vi "Output Message.vi"(0 "Message Expression in":string, 1 "Sequence Context In":refnum<k7>, 5 "Category Expression in":string, 7 "Severity Expression in":string, 9 "Message Severity in":u16(ring) caption="Message Severity" items=["Information", "Warning", "Error"], 11 "Use Severity Expression ? in":bool) -> (4 "Message Expression out":string, 6 "Category Expression out":string, 8 "Severity Expression out":string, 10 "Message Severity out":u16(ring) caption="Message Severity" items=["Information", "Warning", "Error"], 14 "error out":errorcluster, 15 "Use Severity Expression ? out":bool)   [LabVIEW 2020]
uses:
  <vilib>/addons/TestStand/_TSUtility.llb/TestStand - Start Modal Dialog (Sequence Context).vi
  <vilib>/addons/TestStand/_TSUtility.llb/TestStand - End Modal Dialog (Sequence Context).vi
panel:
  in  "Severity Option":T1(tab)
  in  "Message Severity":refnum<k7>(container)
  in  "Cancel":bool
  in  "OK":bool
  in  "Message Category":refnum<k7>(container)
  in  "Message String":refnum<k7>(container)
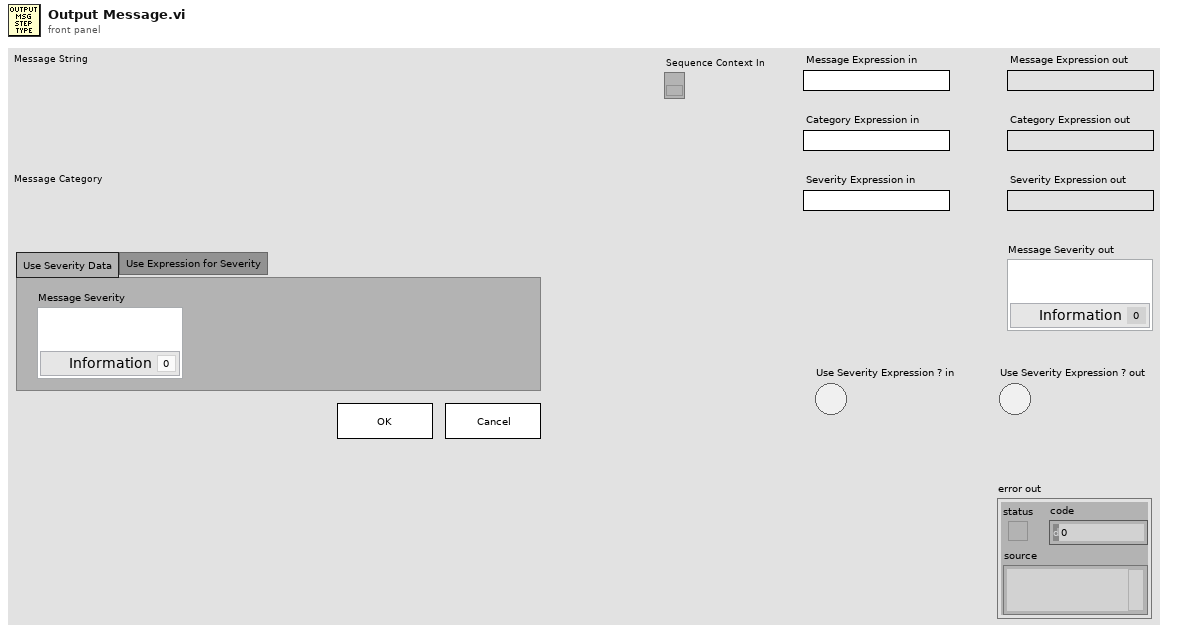
[diagram p1: front panel]
types:
  T1 = enum32{"Use Severity Data", "Use Expression for Severity"}
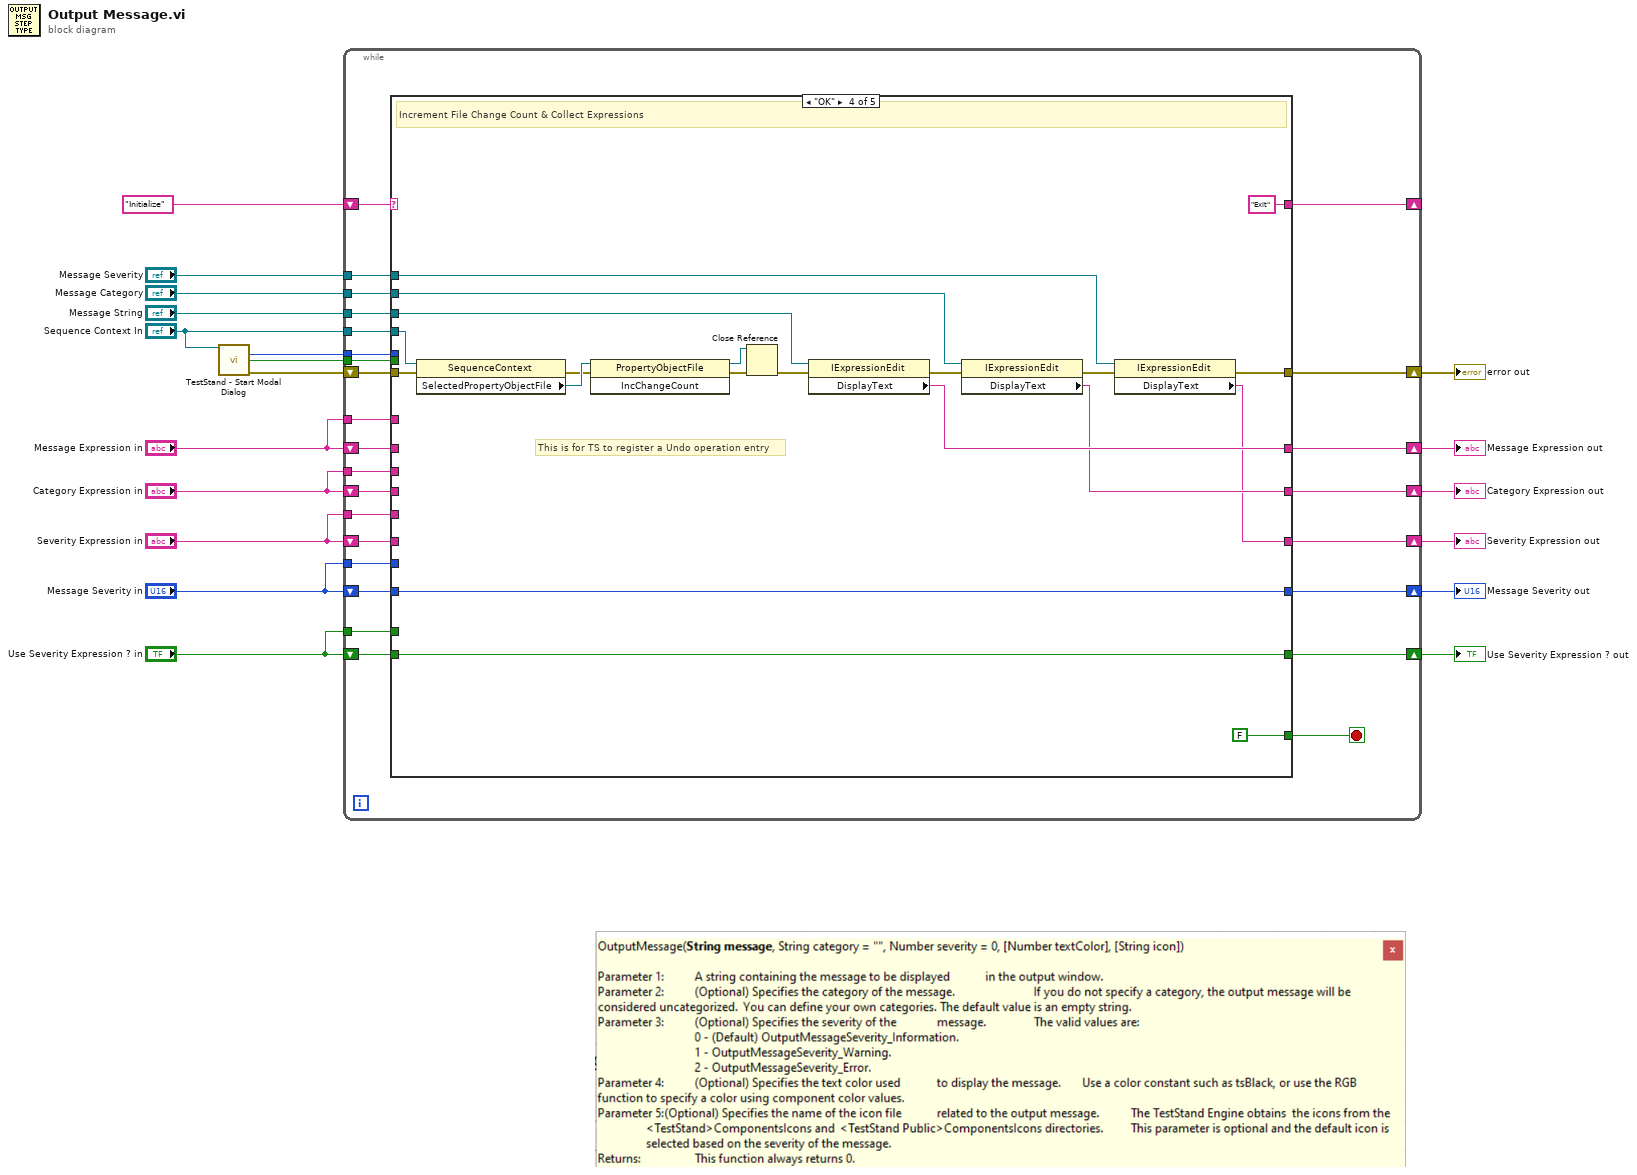
[diagram p0: block diagram]
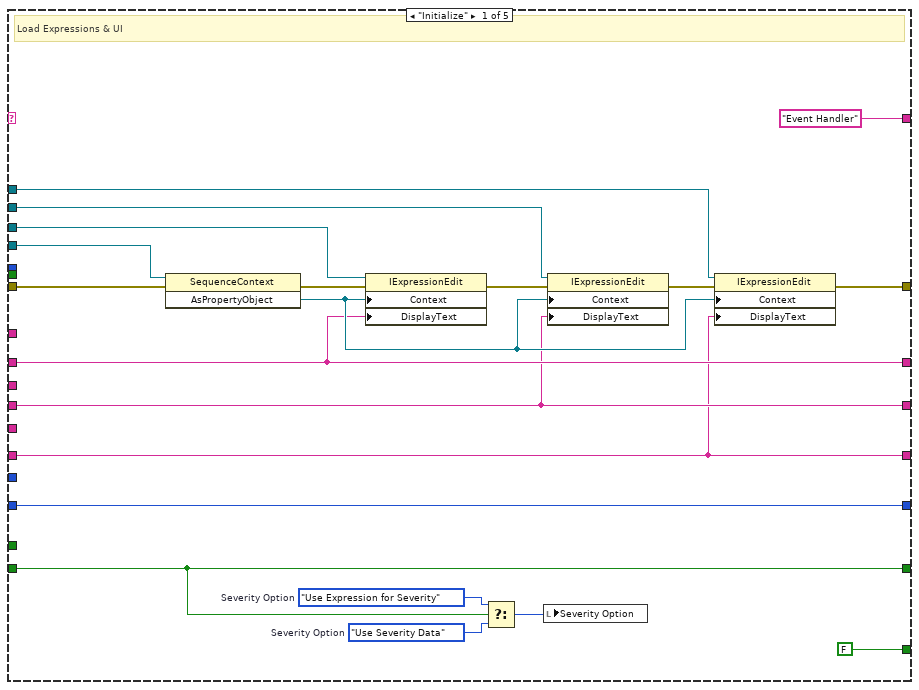
[diagram p2: hidden frame]
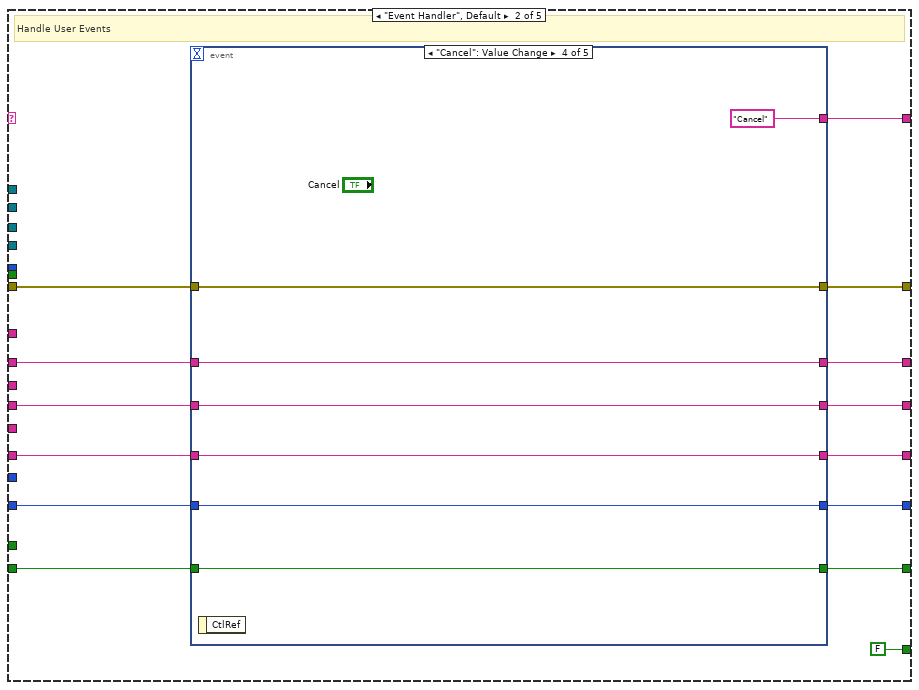
[diagram p3: hidden frame]
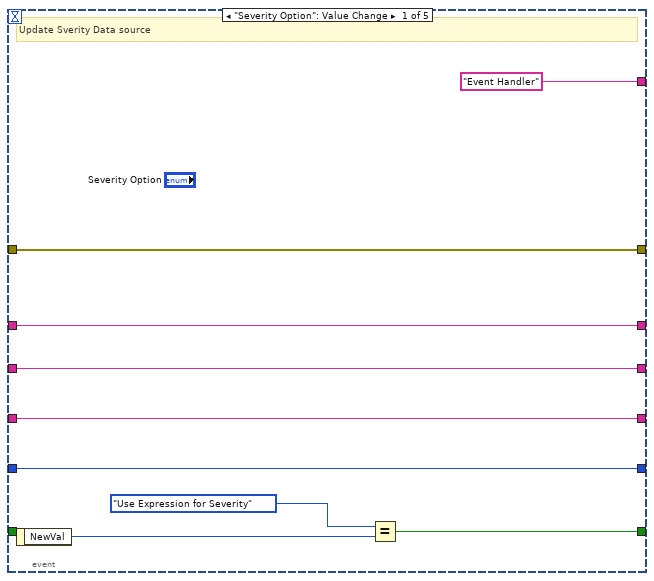
[diagram p4: hidden frame]
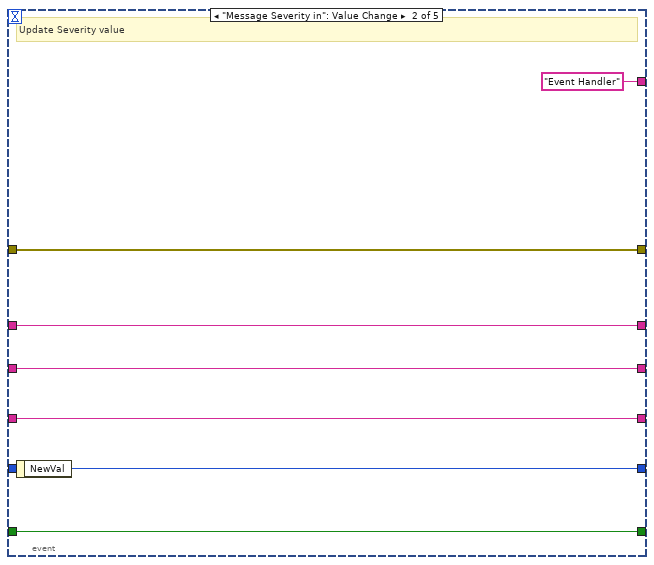
[diagram p5: hidden frame]
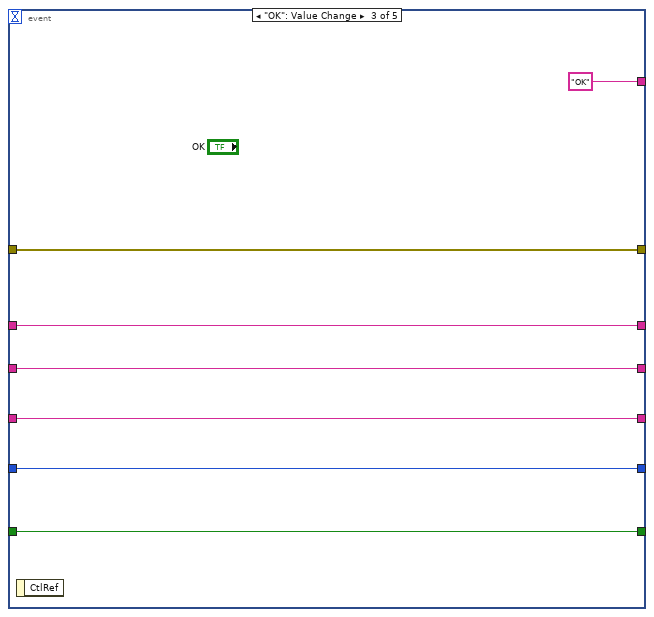
[diagram p6: hidden frame]
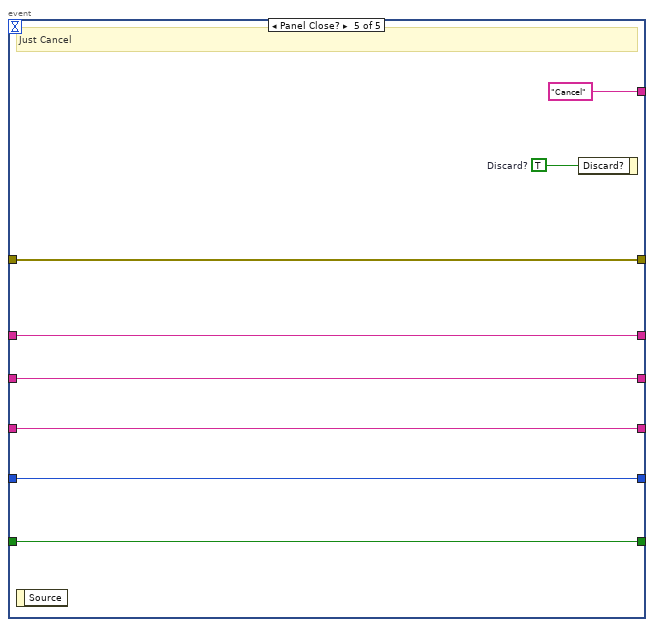
[diagram p7: hidden frame]
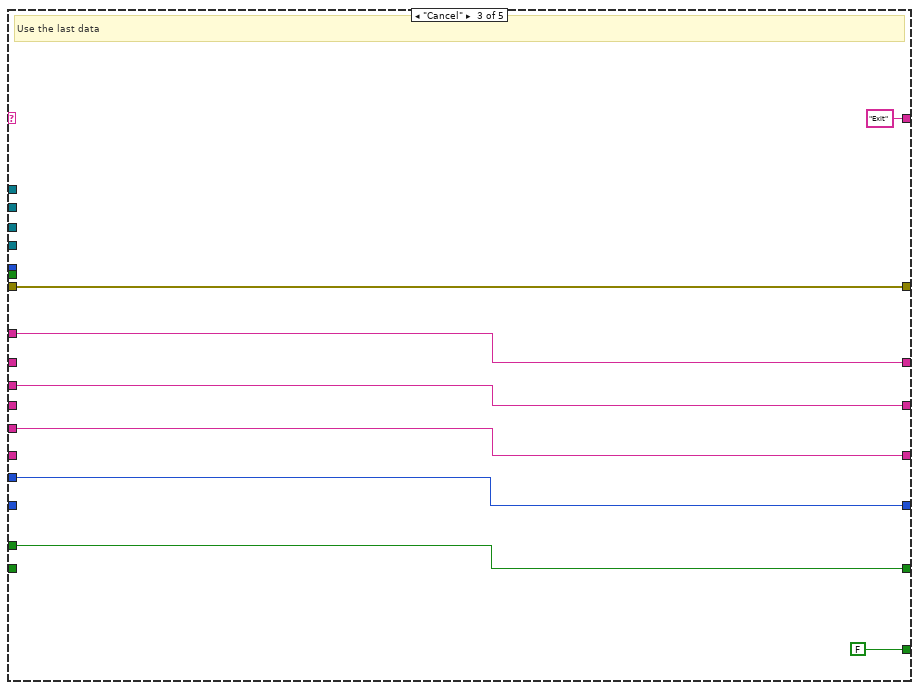
[diagram p8: hidden frame]
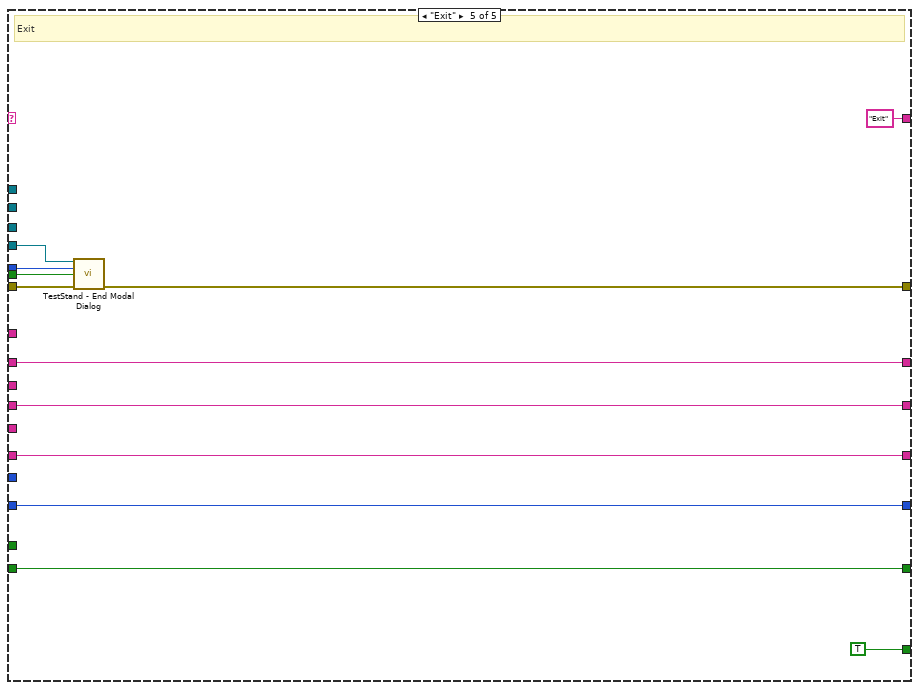
[diagram p9: hidden frame]
diagram:
  n1 = call-poly <vilib>:"TestStand - Start Modal Dialog.vi"("Sequence Context In"="Sequence Context In") -> ("Modal ID"=w2:i32, "VI Originally Open"=w1:bool, "error out"=w4:errorcluster)  [unwired: 10 in, 2 out]
  n2 = while {
    tunnel: "Sequence Context In" -> [w45]
    tunnel: "Message String" -> [w44]
    tunnel: "Message Category" -> [w42]
    tunnel: "Message Severity" -> [w39]
    shift-right: [w36] -> _
    shift-left: "Initialize" -> [w37]
    shift-right: [w34] -> w15
    shift-left: w4 -> [w35]
    shift-right: [w33] -> w10
    shift-left: "Message Expression in" -> [w43]
    shift-right: [w32] -> w9
    shift-left: "Category Expression in" -> [w41]
    shift-right: [w31] -> w6
    shift-left: "Severity Expression in" -> [w40]
    shift-right: [w29] -> w5
    shift-left: "Use Severity Expression ? in" -> [w38]
    tunnel: "Message Expression in" -> [w28]
    tunnel: "Category Expression in" -> [w27]
    tunnel: "Severity Expression in" -> [w26]
    tunnel: "Use Severity Expression ? in" -> [w25]
    tunnel: "Message Severity in" -> [w23]
    shift-right: [w22] -> w8
    shift-left: "Message Severity in" -> [w24]
    tunnel: w2 -> [w21]
    tunnel: w1 -> [w20]
    stop <- w30 stop-if-true
    n3 = case shown="\"OK\"" w37 {
      tunnel: w45 -> [w65 _ _ w132 w153]
      tunnel: w44 -> [w63 _ _ w143 _]
      tunnel: w43 -> [w51 w79 _ _ w148]
      tunnel: w42 -> [w61 _ _ w138 _]
      tunnel: w41 -> [w50 w78 _ _ w147]
      tunnel: w40 -> [w49 w77 _ _ w146]
      tunnel: w39 -> [w58 _ _ w139 _]
      tunnel: [w57 w70 w118 w135 w149] -> w34
      tunnel: w38 -> [w47 w72 _ w133 w154]
      tunnel: ["Event Handler" w68 "Exit" "Exit" "Exit"] -> w36
      tunnel: w35 -> [w52 w69 w118 w127 w152]
      tunnel: [w51 w76 w125 w142 w148] -> w33
      tunnel: [w50 w75 w124 w137 w147] -> w32
      tunnel: [w49 w74 w123 w136 w146] -> w31
      tunnel: [FALSE FALSE FALSE FALSE TRUE] -> w30
      tunnel: [w47 w71 w122 w133 w154] -> w29
      tunnel: w28 -> [_ _ w125 _ _]
      tunnel: w27 -> [_ _ w124 _ _]
      tunnel: w26 -> [_ _ w123 _ _]
      tunnel: w25 -> [_ _ w122 _ _]
      tunnel: w24 -> [w46 w67 _ w134 w155]
      tunnel: w23 -> [_ _ w119 _ _]
      tunnel: [w46 w66 w119 w134 w155] -> w22
      tunnel: w21 -> [_ _ _ _ w151]
      tunnel: w20 -> [_ _ _ _ w150]
      frame "Initialize" {
        w55 = T1."Use Severity Data"  # Severity Option
        w56 = T1."Use Expression for Severity"  # Severity Option
        # "Load Expressions & UI"
        n4 = invoke class="SequenceContext" method="AsPropertyObject"(reference=w65, error in=w52) -> (error out=w64:errorcluster, "AsPropertyObject"=w59:refnum<k7>)  [unwired: 1 in, 1 out]
        n5 = property class="IExpressionEdit"(reference=w63, error in=w64, "Context"=w59, "DisplayText"=w51) -> (error out=w62:errorcluster)  [unwired: 1 out]
        n6 = Select(t=w56, s=w47, f=w55) -> (s? t:f=w54:T1)
        n7 = local write "Severity Option"(w54) -> ()
        n8 = property class="IExpressionEdit"(reference=w61, error in=w62, "Context"=w59, "DisplayText"=w50) -> (error out=w60:errorcluster)  [unwired: 1 out]
        n9 = property class="IExpressionEdit"(reference=w58, error in=w60, "Context"=w59, "DisplayText"=w49) -> (error out=w57:errorcluster)  [unwired: 1 out]
      }
      frame "Event Handler", Default {
        # "Handle User Events"
        n10 = event shown="[3] \"Cancel\": Value Change" {
          selector: _ -> [_ _ _ _ _]
          dyn-events: _ -> [_ _ _ _ _]
          timeout: _ -> [_ _ _ _ _]
          tunnel: w79 -> [w88 w95 w102 w109 w117]
          tunnel: w78 -> [w87 w94 w101 w108 w116]
          tunnel: w77 -> [w86 w93 w100 w107 w115]
          tunnel: [w88 w95 w102 w109 w117] -> w76
          tunnel: [w87 w94 w101 w108 w116] -> w75
          tunnel: [w86 w93 w100 w107 w115] -> w74
          tunnel: w72 -> [_ w92 w99 w106 w114]
          tunnel: [w83 w92 w99 w106 w114] -> w71
          tunnel: [w85 w91 w98 w105 w113] -> w70
          tunnel: w69 -> [w85 w91 w98 w105 w113]
          tunnel: ["Event Handler" "Event Handler" "OK" "Cancel" "Cancel"] -> w68
          tunnel: w67 -> [w80 _ w96 w103 w111]
          tunnel: [w80 w90 w96 w103 w111] -> w66
          event "Severity Option": Value Change {
            # "Update Sverity Data source"
            n11 = event-data() -> ("NewVal"=w84:T1)  [unwired: 1 in]
            n12 = Equal?(x=T1."Use Expression for Severity", y=w84) -> (x = y?=w83:bool)
          }
          event "Message Severity in": Value Change {
            # "Update Severity value"
            n13 = event-data() -> ("NewVal"=w90:u16)  [unwired: 1 in]
          }
          event "OK": Value Change {
            n14 = event-data() -> ()  [unwired: 1 in, 1 out]
          }
          event "Cancel": Value Change {
            n15 = event-data() -> ()  [unwired: 1 in, 1 out]
          }
          event Panel Close? {
            w110 = TRUE  # Discard?
            # "Just Cancel"
            n16 = event-data() -> ()  [unwired: 1 in, 1 out]
            n17 = event-data("Discard?"=w110) -> ()  [unwired: 1 in, 1 out]
          }
        }
      }
      frame "Cancel" {
        # "Use the last data"
      }
      frame "OK" {
        # "This is for TS to register a Undo operation entry"
        # "Increment File Change Count & Collect Expressions"
        n18 = property class="SequenceContext"(reference=w132, error in=w127) -> (error out=w128:errorcluster, "SelectedPropertyObjectFile"=w131:refnum<k7>)  [unwired: 1 out]
        n19 = invoke class="PropertyObjectFile" method="IncChangeCount"(reference=w131, error in=w128) -> (reference out=w129:refnum<k7>, error out=w130:errorcluster)  [unwired: 1 in, 1 out]
        n20 = Close Reference(reference=w129, error in (no error)=w130) -> (error out=w126:errorcluster)
        n21 = property class="IExpressionEdit"(reference=w143, error in=w126) -> (error out=w141:errorcluster, "DisplayText"=w142:string)  [unwired: 1 out]
        n22 = property class="IExpressionEdit"(reference=w138, error in=w141) -> (error out=w140:errorcluster, "DisplayText"=w137:string)  [unwired: 1 out]
        n23 = property class="IExpressionEdit"(reference=w139, error in=w140) -> (error out=w135:errorcluster, "DisplayText"=w136:string)  [unwired: 1 out]
      }
      frame "Exit" {
        # "Exit"
        n24 = call-poly <vilib>:"TestStand - End Modal Dialog.vi"("Sequence Context In"=w153, "Modal ID"=w151, "VI Originally Open"=w150, "error in (no error)"=w152) -> ("error out"=w149:errorcluster)  [unwired: 11 in]
      }
    }
  }
  "error out" <- w15
  "Message Expression out" <- w10
  "Category Expression out" <- w9
  "Message Severity out" <- w8
  "Severity Expression out" <- w6
  "Use Severity Expression ? out" <- w5
